vi "my ao1 one shot on.vi"(0 "device name":tag="Dev1", 1 "stop (T)":bool=TRUE, 2 "timeout (s)":dbl=10.0 format="%0.2f", 7 "voltage out":dbl, 11 "error in":errorcluster) -> (4 "task out":refnum<k21>, 15 "error out":errorcluster)   [LabVIEW 2019]
doc: "Creates, edits, and runs tasks using NI-DAQmx. Refer to the NI-DAQmx Readme for a complete listing of devices NI-DAQmx supports.\n\nWhen you place this Express VI on the block diagram, the DAQ Assistant launches to create a new task. After you create a task, you can double-click the DAQ Assistant Express VI to edit that task. For continuous measurement or generation, place a while loop around the DAQ Assistant Express VI."
uses:
  <vilib>/DAQmx/write.llb/DAQmx Write.vi
  <vilib>/DAQmx/write.llb/DAQmx Write (Analog 1D DBL NChan 1Samp).vi
  <vilib>/DAQmx/create/channels.llb/DAQmx Create Channel (AO-Voltage-Basic).vi
  <vilib>/DAQmx/miscellaneous.llb/DAQmx Fill In Error Info.vi
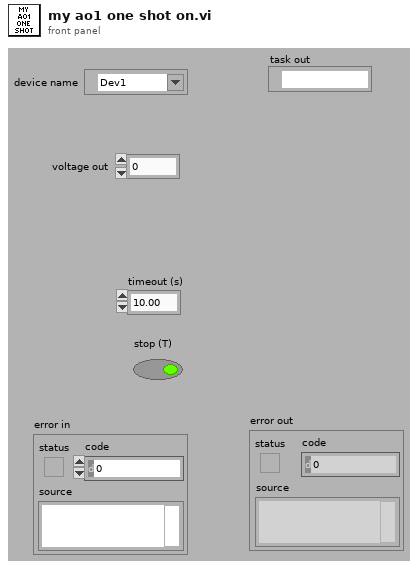
[diagram p1: front panel]
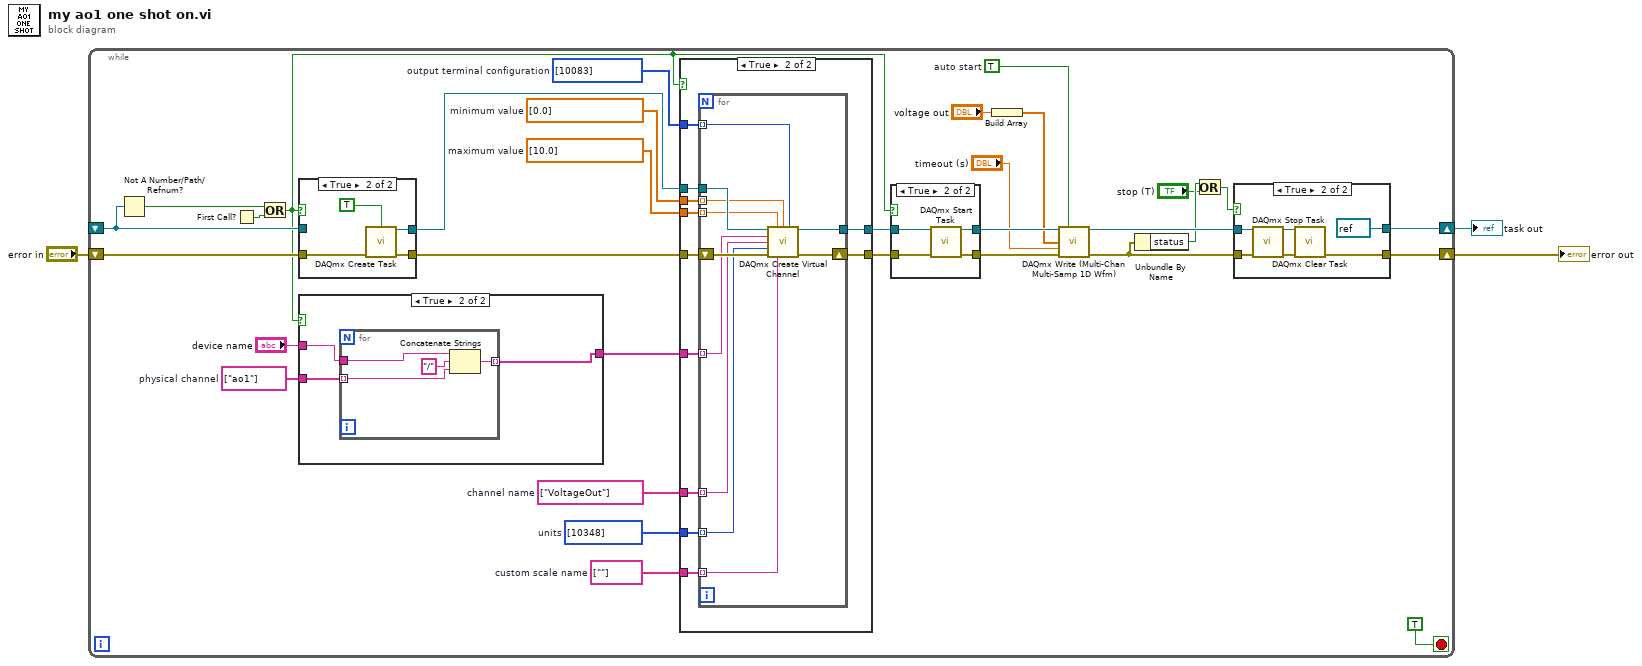
[diagram p0: block diagram]
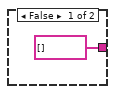
[diagram p5: hidden frame]
diagram:
  n1 = while {
    shift-right: [w13] -> w1
    shift-left: _ -> [w32]
    shift-right: [w11] -> w2
    shift-left: "error in" -> [w33]
    stop <- TRUE stop-if-true
    w6 = TRUE  # auto start
    w20 = i32[] [10083] items=["Default"=-1, "RSE"=10083, "Differential"=10106, "Pseudodifferential"=12529]  # output terminal configuration
    w21 = string[] [""]  # custom scale name
    w22 = i32[] [10348] items=["Volts"=10348, "From Custom Scale"=10065]  # units
    w23 = string[] ["VoltageOut"]  # channel name
    w25 = dbl[] [10.0]  # maximum value
    w26 = dbl[] [0.0]  # minimum value
    w29 = string[] ["ao1"]  # physical channel
    n2 = Not A Number/Path/Refnum?(number/path/refnum=w32) -> (NaN/Path/Refnum?=w31:bool)
    n3 = First Call?() -> (First Call?: T/F=w34:bool)
    n4 = Or(x=w31, y=w34) -> (x .or. y?=w19:bool)
    n5 = case shown="True" w19 {
      tunnel: [w83 w87] -> w28
      tunnel: w32 -> [w83 _]
      tunnel: [w82 w86] -> w27
      tunnel: w33 -> [w82 w84]
      frame False {
      }
      frame True {
        n6 = call <vilib>:"DAQmx Create Task.vi"("auto cleanup"=TRUE, "error in"=w84) -> ("task out"=w87:refnum<k21>, "error out"=w86:errorcluster)  [unwired: 12 in]
      }
    }
    n7 = case shown="True" w19 {
      tunnel: [string[] [] w77] -> w24
      tunnel: "device name" -> [_ w76]
      tunnel: w29 -> [_ w75]
      frame False {
      }
      frame True {
        n8 = for {
          tunnel: [w81] -> w77 mode=indexing
          tunnel: w76 -> [w80]
          tunnel: w75 -> [w78] mode=indexing
          n9 = Concatenate Strings(w80, "/" ("string"), w78) -> (w81:string)
        }
      }
    }
    n10 = case shown="True" w19 {
      tunnel: [w51 w60] -> w18
      tunnel: w28 -> [w51 w62]
      tunnel: [w50 w59] -> w17
      tunnel: w27 -> [w50 w61]
      tunnel: w26 -> [_ w58]
      tunnel: w25 -> [_ w57]
      tunnel: w24 -> [_ w56]
      tunnel: w23 -> [_ w55]
      tunnel: w22 -> [_ w54]
      tunnel: w21 -> [_ w53]
      tunnel: w20 -> [_ w52]
      frame False {
      }
      frame True {
        n11 = for {
          tunnel: w62 -> [w73]
          tunnel: [w71] -> w60
          tunnel: w58 -> [w69] mode=indexing
          tunnel: w57 -> [w68] mode=indexing
          tunnel: w56 -> [w67] mode=indexing
          tunnel: w55 -> [w66] mode=indexing
          tunnel: w54 -> [w65] mode=indexing
          tunnel: w53 -> [w64] mode=indexing
          shift-right: [w70] -> w59
          shift-left: w61 -> [w72]
          tunnel: w52 -> [w63] mode=indexing
          n12 = call-poly <vilib>:"DAQmx Create Virtual Channel.vi"("task in"=w73, "maximum value"=w68, "minimum value"=w69, "output terminal configuration"=w63, "physical channels"=w67, "name to assign"=w66, "units"=w65, "error in"=w72, "custom scale name"=w64) -> ("task out"=w71:refnum<k21>, "error out"=w70:errorcluster)  [unwired: 5 in]
        }
      }
    }
    n13 = case shown="True" w19 {
      tunnel: [w45 w48] -> w16
      tunnel: w18 -> [w45 w49]
      tunnel: [w44 w46] -> w15
      tunnel: w17 -> [w44 w47]
      frame False {
      }
      frame True {
        n14 = call <vilib>:"DAQmx Start Task.vi"("task/channels in"=w49, "error in"=w47) -> ("task out"=w48:refnum<k21>, "error out"=w46:errorcluster)  [unwired: 12 in]
      }
    }
    n15 = Build Array("voltage out") -> (w5:dbl[])
    n16 = call-poly "DAQmx Write (Multi-Chan Multi-Samp 1D Wfm).vi"("task/channels in"=w16, "auto start"=w6, "data"=w5, "timeout"="timeout (s)", "error in"=w15) -> ("task out"=w12:refnum<k21>, "error out"=w10:errorcluster)  [unwired: 8 in, 1 out]
    n17 = Unbundle By Name(w10) -> ("status"=w9:bool)
    n18 = Or(x=w9, y="stop (T)") -> (x .or. y?=w7:bool)
    n19 = case shown="True" w7 {
      tunnel: [w37 refnum<k21> refnum ("task in")] -> w13
      tunnel: w12 -> [w37 w43]
      tunnel: [w36 w40] -> w11
      tunnel: w10 -> [w36 w42]
      frame False {
      }
      frame True {
        n20 = call <vilib>:"DAQmx Stop Task.vi"("task/channels in"=w43, "error in"=w42) -> ("task out"=w39:refnum<k21>, "error out"=w41:errorcluster)  [unwired: 12 in]
        n21 = call <vilib>:"DAQmx Clear Task.vi"("task in"=w39, "error in"=w41) -> ("error out"=w40:errorcluster)  [unwired: 13 in]
      }
    }
  }
  "error out" <- w2
  "task out" <- w1
